vi "Expand.vi"(8 "error in (no error)":errorcluster, 10 "IB_Tree.lvclass":refnum<class "IB_Tree.lvclass">, 11 "IB_TreeRootItem in":refnum<class "IB_Tree_Item_Proj_Container.lvclass">) -> (0 "error out":errorcluster, 2 "first expansion?":bool, 3 "IB_TreeRootItem out":refnum<class "IB_Tree_Item_Proj_Container.lvclass">)   [LabVIEW 2020, in "IB_Tree_Item_Proj_Container.lvclass"]
uses:
  <vilib>/AppBuilder/IB_Classes/Tree_Item_Proj_Container/IB_Tree_Item_Proj_Container.lvclass
  <vilib>/AppBuilder/IB_Classes/Tree_Item_Proj_Container/IB_Tree_Item_Proj_Container.lvclass/IB_Tree_Item_Proj_Container.ctl
  <vilib>/AppBuilder/IB_Classes/Tree/IB_Tree.lvclass
  <vilib>/AppBuilder/IB_Classes/Tree_Item/IB_Tree_Item.lvclass
  e:/builds/penguin/labview/branches/2020/dev/dist/vi.lib/AppBuilder/IB_Classes/Tree_Item_Proj/IB_Tree_Item_Proj.lvclass
  e:/builds/penguin/labview/branches/2020/dev/dist/vi.lib/AppBuilder/IB_Classes/Tree_Item/IB_Tree_Item.lvclass
  e:/builds/penguin/labview/branches/2020/dev/dist/vi.lib/AppBuilder/IB_Classes/Tree_Item_Proj_Container/IB_Tree_Item_Proj_Container.lvclass
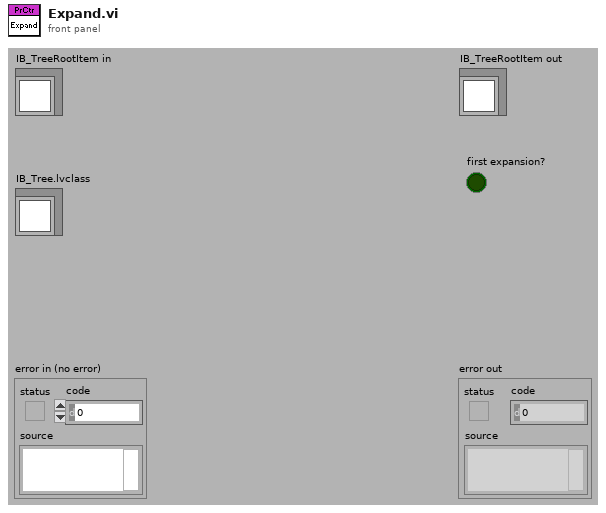
[diagram p1: front panel]
types:
  T1 = typedef "IB_Tree_Item.ctl" = cluster{"symbol index":i32, "child tag":string, "parentTag":string, "left cell name":string}
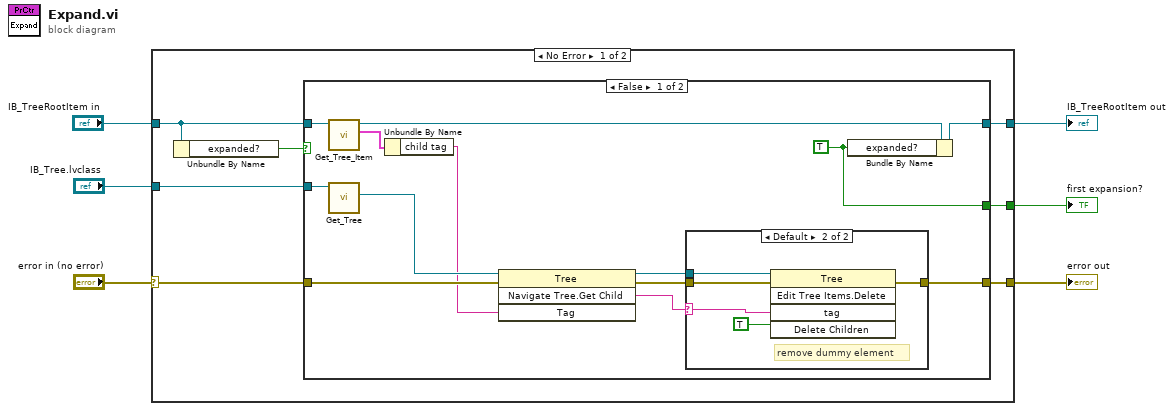
[diagram p0: block diagram]
diagram:
  n1 = case shown="No Error" "error in (no error)" {
    selector: "error in (no error)" -> [w10 w36]
    tunnel: [w9 w36] -> w5
    tunnel: "IB_TreeRootItem in" -> [w11 w35]
    tunnel: "IB_Tree.lvclass" -> [w13 _]
    tunnel: [w8 w35] -> w2
    tunnel: [w7 _] -> w4
    frame No Error {
      n2 = Unbundle By Name(w11) -> ("expanded?"=w12:bool)
      n3 = case shown="False" w12 {
        tunnel: w13 -> [w26 _]
        tunnel: w11 -> [w25 w34]
        tunnel: w10 -> [w17 w33]
        tunnel: [w21 w33] -> w9
        tunnel: [w22 w34] -> w8
        tunnel: [w20 _] -> w7
        frame False {
          w20 = TRUE ("data.previewed?")
          n4 = call <vilib>:"Get_Tree_Item.vi"("IB_TreeItem in"=w25) -> ("data"=w24:T1, "IB_TreeItem out"=w23:refnum<class "IB_Tree_Item_Proj_Container.lvclass">)  [unwired: 8 in, 1 out]
          n5 = call <vilib>:"Get_Tree.vi"("IB_Tree in"=w26) -> ("ctl"=w19:refnum<vi>)  [unwired: 8 in, 2 out]
          n6 = Unbundle By Name(w24) -> ("child tag"=w15:string)
          n7 = invoke class="Tree" method="Navigate Tree.Get Child"(reference=w19, error in=w17, "Tag"=w15) -> (reference out=w18:refnum<vi>, error out=w16:errorcluster, "Navigate Tree:Get Child"=w14:string)  [unwired: 1 in, 1 out]
          n8 = case shown="Default" w14 {
            selector: w14 -> [_ w28]
            tunnel: [w27 w31] -> w21
            tunnel: w18 -> [_ w30]
            tunnel: w16 -> [w27 w29]
            frame "" {
            }
            frame Default {
              # "remove dummy element"
              n9 = invoke class="Tree" method="Edit Tree Items.Delete"(reference=w30, error in=w29, "tag"=w28, "Delete Children"=TRUE ("Delete Children?")) -> (error out=w31:errorcluster)  [unwired: 1 in, 4 out]
            }
          }
          n10 = Bundle By Name(cluster=w23, "expanded?"=w20) -> (w22:refnum<class "IB_Tree_Item_Proj_Container.lvclass">)
        }
        frame True {
        }
      }
    }
    frame Error {
    }
  }
  "error out" <- w5
  "IB_TreeRootItem out" <- w2
  "first expansion?" <- w4
